vi "Separate particles.vi"(11 "Good particles in 3":T1(array[cluster])) -> (2 "|_ particles":T1(array[cluster]), 3 "_| particles":T1(array[cluster]))   [LabVIEW 2015]
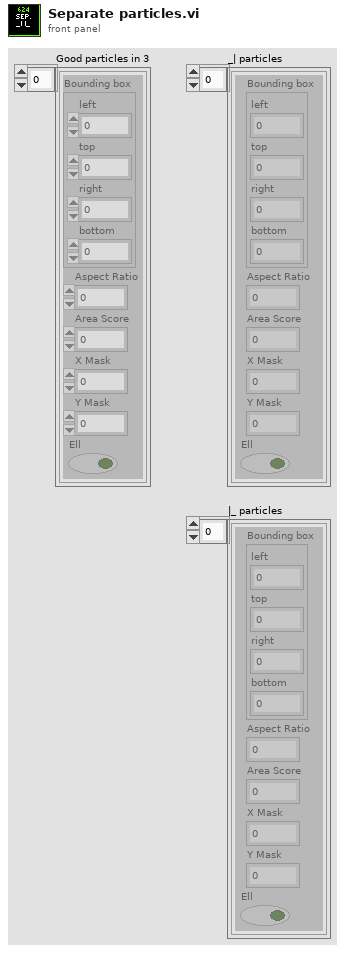
[diagram p1: front panel]
types:
  T1 = cluster{"Bounding box":cluster{"left":dbl, "top":dbl, "right":dbl, "bottom":dbl}, "Aspect Ratio":dbl, "Area Score":dbl, "X Mask":dbl, "Y Mask":dbl, "Ell":bool}[]
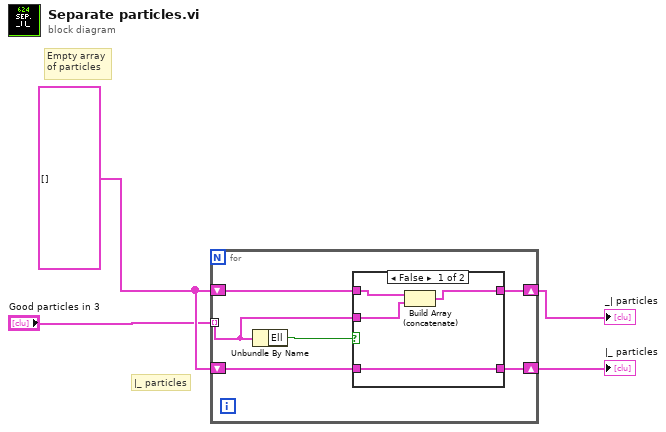
[diagram p0: block diagram]
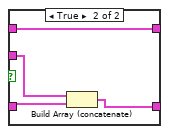
[diagram p2: hidden frame]
diagram:
  w2 = T1 [] ("Good particles in")
  # "|_ particles"
  # "Empty array\nof particles"
  n1 = for {
    tunnel: "Good particles in 3" -> [w6] mode=indexing
    shift-right: [w7] -> w3
    shift-left: w2 -> [w9]
    shift-right: [w5] -> w4
    shift-left: w2 -> [w8]
    n2 = Unbundle By Name(w6) -> ("Ell"=w10:bool)
    n3 = case shown="False" w10 {
      tunnel: w9 -> [w14 w18]
      tunnel: w8 -> [w11 w16]
      tunnel: [w13 w18] -> w7
      tunnel: w6 -> [w12 w17]
      tunnel: [w11 w15] -> w5
      frame False {
        n4 = Build Array (concatenate)(w14, w12) -> (w13:T1)
      }
      frame True {
        n5 = Build Array (concatenate)(w17, w16) -> (w15:T1)
      }
    }
  }
  "|_ particles" <- w4
  "_| particles" <- w3
